vi "Initialize Instrument.vi"(8 "error in (no error)":errorcluster, 10 "Reset":bool, 11 "VNA-Ag87xx in":refnum<class "VNA-Ag87xx.lvclass">) -> (0 "error out":errorcluster, 3 "VNA-Ag87xx out":refnum<class "VNA-Ag87xx.lvclass">)   [LabVIEW 2020, in "VNA-Ag87xx.lvclass"]
uses:
  VNA-Ag87xx.lvclass
  C:/Sandbox/RF Bench/Source Code/WiSpry Test Framework/Instruments/Instrument.lvclass
  C:/Sandbox/RF Bench/Source Code/WiSpry Test Framework/Instruments/Vector Network Analyzer/Vector Network Analyzer.lvclass
  <vilib>/Instr/_visa.llb/VISA Open Access Mode.ctl
  Instrument.lvclass/Instrument.ctl
  Vector Network Analyzer.lvclass/Vector Network Analyzer.ctl
  Instrument.lvclass
  Vector Network Analyzer.lvclass
  <instrlib>/Agilent 87XX Series/Agilent 87XX Series.lvlib
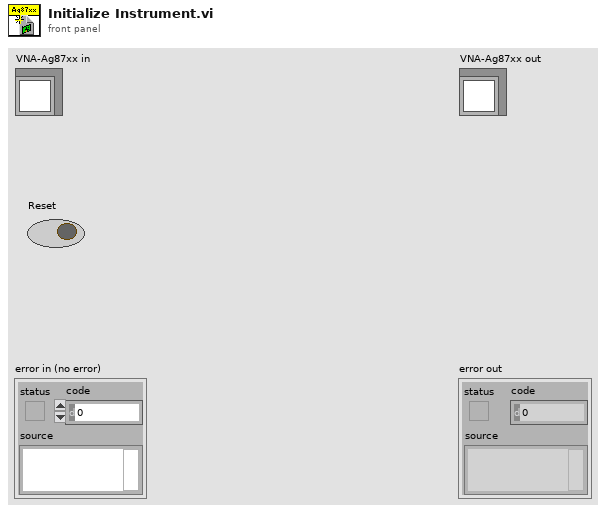
[diagram p1: front panel]
types:
  T1 = typedef "VISA Open Access Mode.ctl" = u32
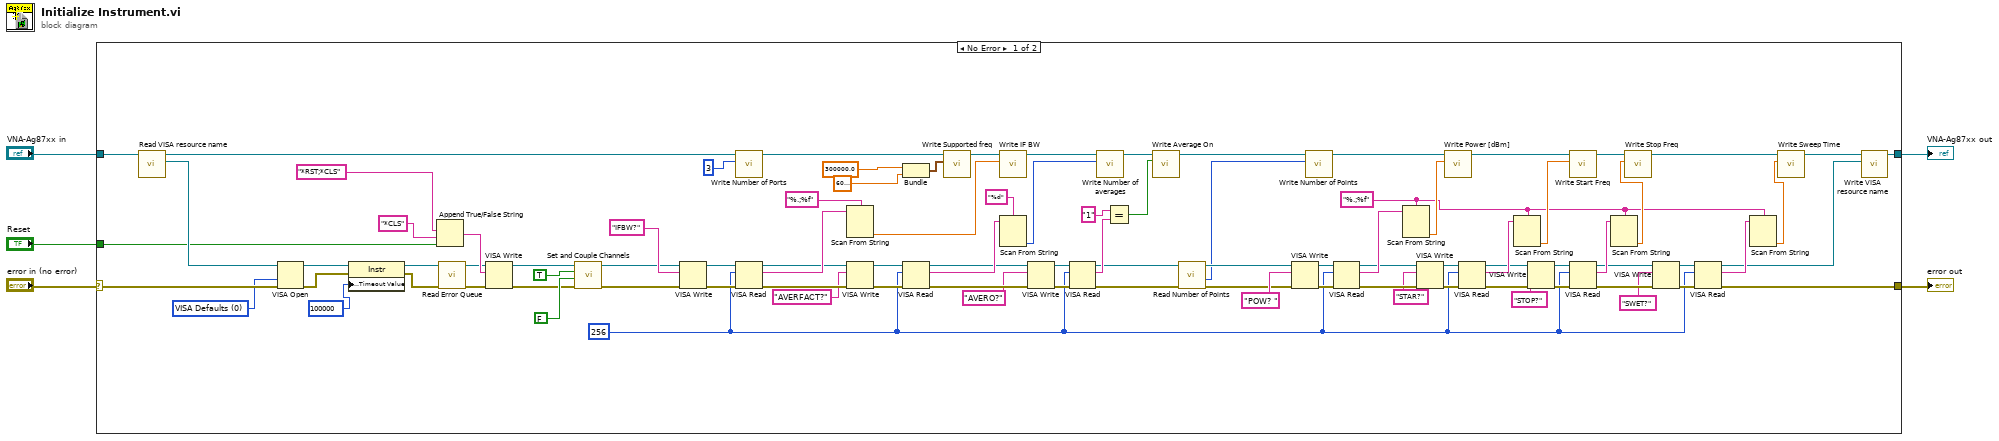
[diagram p0: block diagram]
diagram:
  n1 = case shown="No Error" "error in (no error)" {
    selector: "error in (no error)" -> [w98 w100]
    tunnel: "VNA-Ag87xx in" -> [w99 w101]
    tunnel: [w23 w100] -> w2
    tunnel: [w70 w101] -> w1
    tunnel: "Reset" -> [w21 _]
    frame No Error {
      w25 = "%.;%f" ("format string")
      w29 = u32 256 ("byte count")
      w96 = T1 0 items=["VISA Defaults"=0, "Exclusive Lock"=1, "Load Configured Settings"=4] ("Access Mode")
      n2 = call "Read VISA resource name.vi"("Instrument in"=w99) -> ("VISA resource name"=w97:refnum<visa-resource-name>, "Instrument out"=w92:refnum<class "VNA-Ag87xx.lvclass">)  [unwired: 9 in]
      n3 = VISA Open(access mode=w96, error in (no error)=w98, VISA resource name=w97) -> (VISA resource name=w94:refnum<visa-resource-name>, error out=w93:errorcluster)  [unwired: 2 in]
      n4 = property class="Instr"(reference=w94, error in=w93, "General Settings:Timeout Value"=u32 100000) -> (reference out=w15:refnum<visa-resource-name>, error out=w14:errorcluster)
      n5 = Append True/False String(1:w21, 2:"*CLS" ("false string"), 3:"*RST;*CLS" ("Default Setup String")) -> (0:w89:string)  [unwired: 1 in]
      n6 = call <instrlib>:"Read Error Queue.vi"("error in (no error)"=w14, "VISA resource name"=w15) -> ("error out"=w13:errorcluster, "VISA resource name out"=w12:refnum<visa-resource-name>)  [unwired: 6 in, 2 out]
      n7 = VISA Write(VISA resource name=w12, write buffer=w89, error in (no error)=w13) -> (VISA resource name out=w10:refnum<visa-resource-name>, error out=w9:errorcluster)  [unwired: 1 out]
      n8 = call <instrlib>:"Set and Couple Channels.vi"("error in (no error)"=w9, "channels coupled (F : uncoupled)"=FALSE, "active channel (T : CH1)"=TRUE, "VISA resource name"=w10) -> ("error out"=w8:errorcluster, "VISA resource name out"=w7:refnum<visa-resource-name>)  [unwired: 6 in]
      n9 = VISA Write(VISA resource name=w7, write buffer="IFBW?", error in (no error)=w8) -> (VISA resource name out=w77:refnum<visa-resource-name>, error out=w75:errorcluster)  [unwired: 1 out]
      n10 = call "Write Number of Ports.vi"("Number of Ports"=3, "Vector Network Analyzer in"=w92) -> ("Vector Network Analyzer out"=w88:refnum<class "VNA-Ag87xx.lvclass">)  [unwired: 9 in]
      n11 = VISA Read(VISA resource name=w77, byte count=w29, error in (no error)=w75) -> (VISA resource name out=w68:refnum<visa-resource-name>, read buffer=w73:string, error out=w67:errorcluster)  [unwired: 1 out]
      n12 = Scan From String(format string="%.;%f", input string=w73) -> (output 1=w72:dbl)  [unwired: 3 in, 3 out]
      n13 = VISA Write(VISA resource name=w68, write buffer="AVERFACT?", error in (no error)=w67) -> (VISA resource name out=w65:refnum<visa-resource-name>, error out=w69:errorcluster)  [unwired: 1 out]
      n14 = Bundle(300000.0, 6000000000.0) -> (w87:cluster{dbl, dbl})  [unwired: 1 in]
      n15 = VISA Read(VISA resource name=w65, byte count=w29, error in (no error)=w69) -> (VISA resource name out=w59:refnum<visa-resource-name>, read buffer=w64:string, error out=w58:errorcluster)  [unwired: 1 out]
      n16 = call "Write Supported freq.vi"("Supported freq"=w87, "Vector Network Analyzer in"=w88) -> ("Vector Network Analyzer out"=w71:refnum<class "VNA-Ag87xx.lvclass">)  [unwired: 9 in]
      n17 = call "Write IF BW.vi"("IF BW"=w72, "Vector Network Analyzer in"=w71) -> ("Vector Network Analyzer out"=w86:refnum<class "VNA-Ag87xx.lvclass">)  [unwired: 9 in]
      n18 = Scan From String(format string="%d", input string=w64) -> (output 1=w62:i32)  [unwired: 3 in, 3 out]
      n19 = VISA Write(VISA resource name=w59, write buffer="AVERO?", error in (no error)=w58) -> (VISA resource name out=w61:refnum<visa-resource-name>, error out=w60:errorcluster)  [unwired: 1 out]
      n20 = VISA Read(VISA resource name=w61, byte count=w29, error in (no error)=w60) -> (VISA resource name out=w20:refnum<visa-resource-name>, read buffer=w56:string, error out=w19:errorcluster)  [unwired: 1 out]
      n21 = call "Write Number of averages.vi"("Number of averages"=w62, "Vector Network Analyzer in"=w86) -> ("Vector Network Analyzer out"=w85:refnum<class "VNA-Ag87xx.lvclass">)  [unwired: 9 in]
      n22 = Equal?(x="1", y=w56) -> (x = y?=w54:bool)
      n23 = call "Write Average On.vi"("Average On"=w54, "Vector Network Analyzer in"=w85) -> ("Vector Network Analyzer out"=w84:refnum<class "VNA-Ag87xx.lvclass">)  [unwired: 9 in]
      n24 = call <instrlib>:"Read Number of Points.vi"("error in (no error)"=w19, "VISA resource name"=w20) -> ("error out"=w18:errorcluster, "num points"=w16:i32, "VISA resource name out"=w17:refnum<visa-resource-name>)  [unwired: 7 in]
      n25 = VISA Write(VISA resource name=w17, write buffer="POW? ", error in (no error)=w18) -> (VISA resource name out=w53:refnum<visa-resource-name>, error out=w52:errorcluster)  [unwired: 1 out]
      n26 = call "Write Number of Points.vi"("Number of Points"=w16, "Vector Network Analyzer in"=w84) -> ("Vector Network Analyzer out"=w83:refnum<class "VNA-Ag87xx.lvclass">)  [unwired: 9 in]
      n27 = VISA Read(VISA resource name=w53, byte count=w29, error in (no error)=w52) -> (VISA resource name out=w46:refnum<visa-resource-name>, read buffer=w50:string, error out=w45:errorcluster)  [unwired: 1 out]
      n28 = Scan From String(format string=w25, input string=w50) -> (output 1=w49:dbl)  [unwired: 3 in, 3 out]
      n29 = VISA Write(VISA resource name=w46, write buffer="STAR?", error in (no error)=w45) -> (VISA resource name out=w47:refnum<visa-resource-name>, error out=w48:errorcluster)  [unwired: 1 out]
      n30 = call "Write Power [dBm].vi"("Power [dBm]"=w49, "Vector Network Analyzer in"=w83) -> ("Vector Network Analyzer out"=w82:refnum<class "VNA-Ag87xx.lvclass">)  [unwired: 9 in]
      n31 = VISA Read(VISA resource name=w47, byte count=w29, error in (no error)=w48) -> (VISA resource name out=w40:refnum<visa-resource-name>, read buffer=w43:string, error out=w39:errorcluster)  [unwired: 1 out]
      n32 = Scan From String(format string=w25, input string=w43) -> (output 1=w42:dbl)  [unwired: 3 in, 3 out]
      n33 = VISA Write(VISA resource name=w40, write buffer="STOP?", error in (no error)=w39) -> (VISA resource name out=w41:refnum<visa-resource-name>, error out=w37:errorcluster)  [unwired: 1 out]
      n34 = call "Write Start Freq.vi"("Start Freq"=w42, "Vector Network Analyzer in"=w82) -> ("Vector Network Analyzer out"=w81:refnum<class "VNA-Ag87xx.lvclass">)  [unwired: 9 in]
      n35 = VISA Read(VISA resource name=w41, byte count=w29, error in (no error)=w37) -> (VISA resource name out=w32:refnum<visa-resource-name>, read buffer=w35:string, error out=w31:errorcluster)  [unwired: 1 out]
      n36 = Scan From String(format string=w25, input string=w35) -> (output 1=w36:dbl)  [unwired: 3 in, 3 out]
      n37 = call "Write Stop Freq.vi"("Stop Freq"=w36, "Vector Network Analyzer in"=w81) -> ("Vector Network Analyzer out"=w28:refnum<class "VNA-Ag87xx.lvclass">)  [unwired: 9 in]
      n38 = VISA Write(VISA resource name=w32, write buffer="SWET?", error in (no error)=w31) -> (VISA resource name out=w33:refnum<visa-resource-name>, error out=w34:errorcluster)  [unwired: 1 out]
      n39 = VISA Read(VISA resource name=w33, byte count=w29, error in (no error)=w34) -> (VISA resource name out=w22:refnum<visa-resource-name>, read buffer=w26:string, error out=w23:errorcluster)  [unwired: 1 out]
      n40 = Scan From String(format string=w25, input string=w26) -> (output 1=w24:dbl)  [unwired: 3 in, 3 out]
      n41 = call "Write Sweep Time.vi"("Sweep Time"=w24, "Vector Network Analyzer in"=w28) -> ("Vector Network Analyzer out"=w27:refnum<class "VNA-Ag87xx.lvclass">)  [unwired: 9 in]
      n42 = call "Write VISA resource name.vi"("VISA resource name"=w22, "Instrument in"=w27) -> ("Instrument out"=w70:refnum<class "VNA-Ag87xx.lvclass">)  [unwired: 9 in]
    }
    frame Error {
    }
  }
  "error out" <- w2
  "VNA-Ag87xx out" <- w1
